vi "Arduino Target Test.vi"() -> ()   [LabVIEW 2014, in "ESP8266 WiFi Wrapper.lvlib"]
uses:
  ESP8266 WiFi Wrapper.lvlib
panel:
  out "Error Out":errorcluster
  in  "Error In":errorcluster
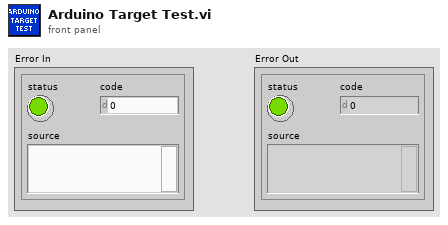
[diagram p1: front panel]
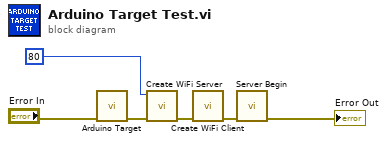
[diagram p0: block diagram]
diagram:
  n1 = call "Arduino Target.vi"("Error In"="Error In") -> ("Error Out"=w3:errorcluster)  [unwired: 10 in]
  n2 = call "Create WiFi Server.vi"("Error In"=w3, "Listen Port"=u8 80) -> ("Error Out"=w2:errorcluster)  [unwired: 9 in]
  n3 = call "Create WiFi Client.vi"("Error In"=w2) -> ("Error Out"=w6:errorcluster)  [unwired: 10 in]
  n4 = call "Server Begin.vi"("Error In"=w6) -> ("Error Out"=→"Error Out":errorcluster)  [unwired: 10 in]
